vi "Calibrate DO Sensor.vi"(6 "Initialize/Close?":bool, 7 "Calibration Standard":dbl, 8 "Error In (No Error)":errorcluster, 9 "Calibrate":bool=TRUE, 10 "Sensor Address In":string="0", 11 "RS232 Port In":refnum<visa-resource-name>="COM11") -> (0 "Error Out":errorcluster, 1 "Sensor Calibrate Response":bool, 2 "Address Out":string, 3 "RS232 Port Out":refnum<visa-resource-name>)   [LabVIEW 2016]
doc: "Sends an SDI-12 Send Identification Command, and returns the various attributes from the sensor's response.\n\nThe total size by the sensor must be 22-35 in size (inclusive), or this VI will return an error."
uses:
  SDI-12/SDI-12.lvlib
panel:
  out "read buffer":string
  out "output 1":i16
  out "Command":string
  # "(c) 2008 National Instruments.  ALL RIGHTS RESERVED."
  # "The following are required,\nor are optional, for the sensors\nto respond with:"
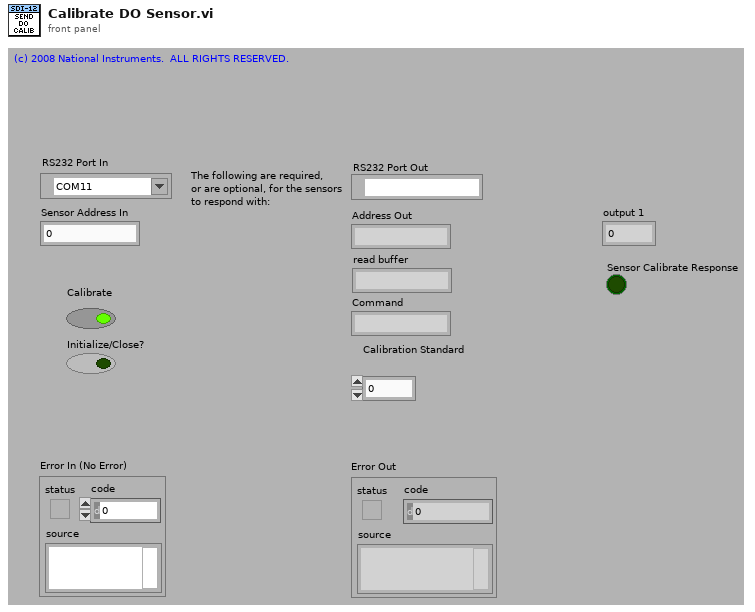
[diagram p1: front panel]
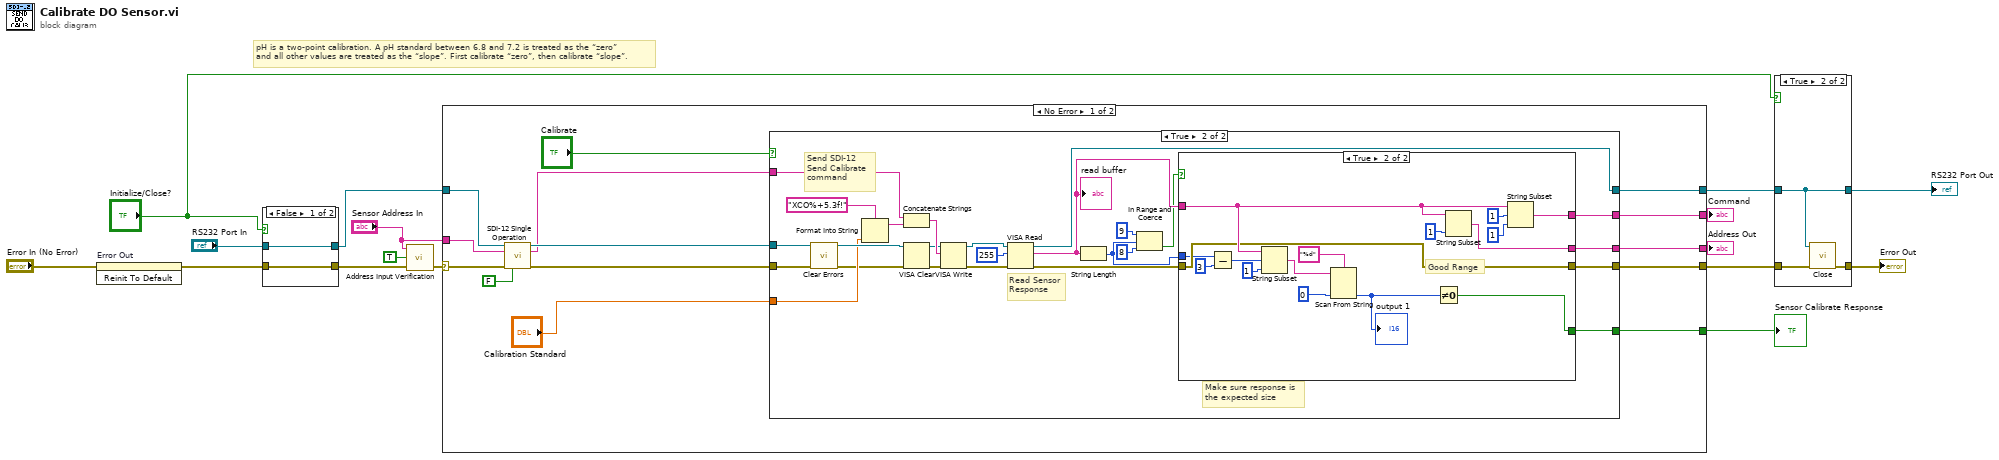
[diagram p0: block diagram]
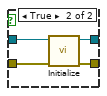
[diagram p3: hidden frame]
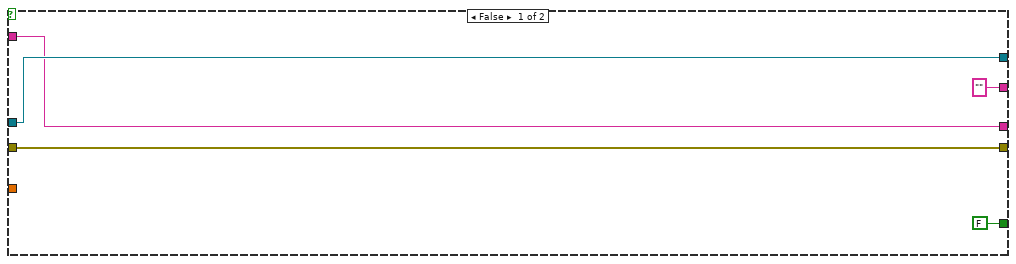
[diagram p4: hidden frame]
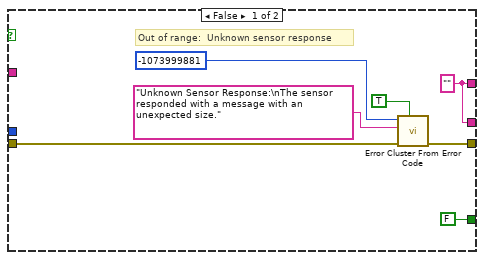
[diagram p5: hidden frame]
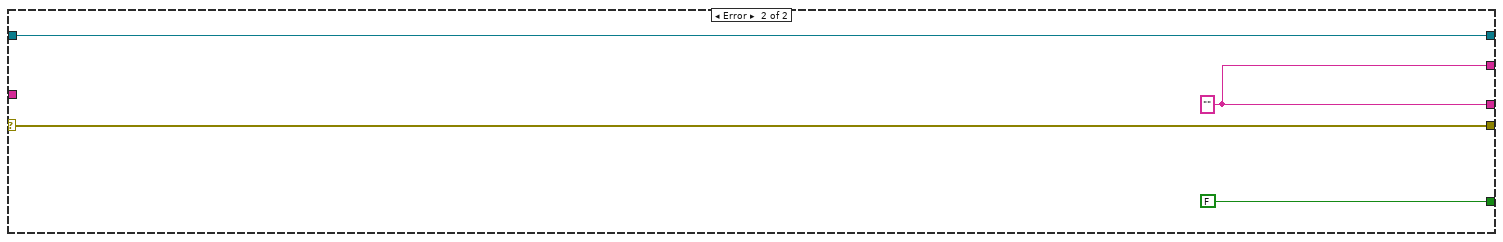
[diagram p6: hidden frame]
diagram:
  # "pH is a two-point calibration. A pH standard between 6.8 and 7.2 is treated as the “zero”\nand all other values are treated as the “slope”. First calibrate “zero”, then calibrate “slope”."
  n1 = invoke on="Error Out" class="Clust (strict)" method="Reinit To Default"(error in="Error In (No Error)") -> (error out=w1:errorcluster)  [unwired: 2 in, 2 out]
  n2 = case shown="False" "Initialize/Close?" {
    tunnel: w1 -> [w18 w22]
    tunnel: [w18 w21] -> w6
    tunnel: "RS232 Port In" -> [w17 w20]
    tunnel: [w17 w19] -> w4
    frame False {
    }
    frame True {
      n3 = call "Initialize.vi"("Error In (No Error)"=w22, "RS232 Port In"=w20) -> ("Error Out"=w21:errorcluster, "RS232 Port Out"=w19:refnum<visa-resource-name>)  [unwired: 8 in]
    }
  }
  n4 = call "Address Input Verification.vi"("Error In (No Error)"=w6, "Error if Bad? (True)"=TRUE ("error if bad? (True)"), "Sensor Address In (a)"="Sensor Address In") -> ("Error Out"=w16:errorcluster)  [unwired: 1 in, 1 out]
  n5 = case shown="No Error" w16 {
    selector: w16 -> [w30 w92]
    tunnel: [w35 w92] -> w10
    tunnel: "Sensor Address In" -> [w26 _]
    tunnel: w4 -> [w28 w91]
    tunnel: [w36 w91] -> w7
    tunnel: [w34 w90] -> w12
    tunnel: [w33 w90] -> w13
    tunnel: [w32 FALSE] -> w11
    frame No Error {
      n6 = call "SDI-12 Single Operation.vi"("RS232 Port In"=w28, "Sensor Address In"=w26, "Error In (No Error)"=w30, "Initialize/Close?"=FALSE) -> ("RS232 Port Out"=w27:refnum<visa-resource-name>, "Address Out"=w25:string, "Error Out"=w29:errorcluster)  [unwired: 7 in, 2 out]
      n7 = case shown="True" "Calibrate" {
        tunnel: w25 -> [w39 w62]
        tunnel: w27 -> [w41 w60]
        tunnel: [w41 w59] -> w36
        tunnel: [w40 w53] -> w35
        tunnel: ["" ("read buffer") w52] -> w34
        tunnel: [w39 w51] -> w33
        tunnel: [FALSE w48] -> w32
        tunnel: w29 -> [w40 w46]
        tunnel: "Calibration Standard" -> [_ w43]
        frame False {
        }
        frame True {
          # "Make sure response is\nthe expected size"
          # "Send SDI-12 \nSend Calibrate \ncommand"
          # "Read Sensor\nResponse"
          n8 = call <vilib>:"Clear Errors.vi"("error in (no error)"=w46) -> ("error out"=w42:errorcluster)  [unwired: 5 in, 1 out]
          n9 = Format Into String(format string="XCO%+5.3f!", w43) -> (resulting string=w49:string)  [unwired: 2 in, 1 out]
          n10 = Concatenate Strings(w62, w49) -> (w61:string)
          n11 = VISA Clear(VISA resource name=w60, error in (no error)=w42) -> (VISA resource name out=w47:refnum<visa-resource-name>, error out=w45:errorcluster)
          n12 = VISA Write(VISA resource name=w47, write buffer=w61, error in (no error)=w45) -> (VISA resource name out=w65:refnum<visa-resource-name>, error out=w64:errorcluster)  [unwired: 1 out]
          n13 = VISA Read(VISA resource name=w65, byte count=u32 255, error in (no error)=w64) -> (VISA resource name out=w59:refnum<visa-resource-name>, read buffer=w55:string, error out=w56:errorcluster)  [unwired: 1 out]
          "read buffer" <- w55
          n14 = String Length(string=w55) -> (length=w44:i32)
          n15 = In Range and Coerce(upper limit=9, x=w44, lower limit=8) -> (In Range?=w54:bool)  [unwired: 1 out]
          n16 = case shown="True" w54 {
            tunnel: w56 -> [w68 w83]
            tunnel: [w69 w83] -> w53
            tunnel: w55 -> [_ w85]
            tunnel: [w67 w81] -> w52
            tunnel: [w67 w80] -> w51
            tunnel: [FALSE w76] -> w48
            tunnel: w44 -> [_ w75]
            frame False {
              w67 = "" ("read buffer")
              # "Out of range:  Unknown sensor response"
              n17 = call <vilib>:"Error Cluster From Error Code.vi"("show call chain? (False)"=TRUE, "error in (no error)"=w68, "error message (\"\")"="Unknown Sensor Response:\nThe sensor responded with a message with an unexpected size." ("error message (\"\")"), "error code (0)"=-1073999881) -> ("error out"=w69:errorcluster)  [unwired: 5 in]
            }
            frame True {
              # "Good Range"
              n18 = Subtract(x=w75, y=3) -> (x-y=w74:i32)
              n19 = String Subset(string=w85, offset (0)=w74, length (rest)=1 ("length (rest)")) -> (substring=w82:string)
              n20 = Scan From String(format string="%d", input string=w82, default 1=i16 0 ("default value 1")) -> (output 1=w77:i16)  [unwired: 2 in, 3 out]
              "output 1" <- w77
              n21 = Not Equal To 0?(x=w77) -> (x != 0?=w76:bool)
              n22 = String Subset(string=w85, length (rest)=1 ("length (rest)")) -> (substring=w80:string)  [unwired: 1 in]
              n23 = String Subset(string=w85, offset (0)=1, length (rest)=1 ("length (rest)")) -> (substring=w81:string)
            }
          }
        }
      }
    }
    frame Error {
      w90 = "" ("read buffer")
    }
  }
  "Command" <- w12
  "Address Out" <- w13
  "Sensor Calibrate Response" <- w11
  n24 = case shown="True" "Initialize/Close?" {
    tunnel: w10 -> [w94 w97]
    tunnel: [w94 w96] -> w9
    tunnel: w7 -> [w93 w95]
    tunnel: [w93 w95] -> w8
    frame False {
    }
    frame True {
      n25 = call "Close.vi"("Error In (No Error)"=w97, "RS232 Port In"=w95) -> ("Error Out"=w96:errorcluster)  [unwired: 9 in]
    }
  }
  "Error Out" <- w9
  "RS232 Port Out" <- w8
